vi "DeadBand.vi"(9 "R In":dbl, 10 "Y In":dbl, 11 "X In":dbl) -> (1 "R Out":dbl, 2 "Y Out":dbl, 3 "X Out":dbl)   [LabVIEW 2015]
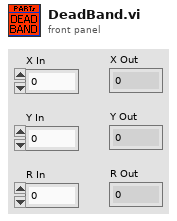
[diagram p1: front panel]
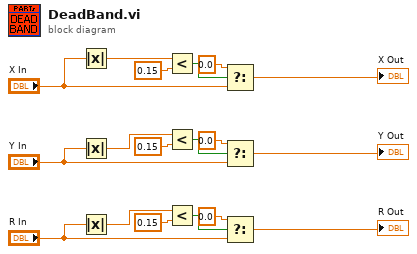
[diagram p0: block diagram]
diagram:
  n1 = Absolute Value(x="X In") -> (abs(x)=w12:dbl)
  n2 = Absolute Value(x="Y In") -> (abs(x)=w8:dbl)
  n3 = Absolute Value(x="R In") -> (abs(x)=w1:dbl)
  n4 = Less?(x=w12, y=0.15) -> (x < y?=w10:bool)
  n5 = Less?(x=w8, y=0.15) -> (x < y?=w6:bool)
  n6 = Less?(x=w1, y=0.15) -> (x < y?=w3:bool)
  n7 = Select(t=0.0, s=w10, f="X In") -> (s? t:f=→"X Out":dbl)
  n8 = Select(t=0.0, s=w6, f="Y In") -> (s? t:f=→"Y Out":dbl)
  n9 = Select(t=0.0, s=w3, f="R In") -> (s? t:f=→"R Out":dbl)
